vi "Sub-VI_Erros-Soma-Sensores.vi"(0 "Boolean 2":bool, 1 "Boolean 3":bool, 2 "Boolean 9":bool, 3 "Boolean 6":bool, 4 "Boolean 4":bool, 5 "Boolean 5":bool, 6 "Boolean 7":bool, 7 "Boolean 8":bool) -> (14 "Boolean":bool)   [LabVIEW 2019]
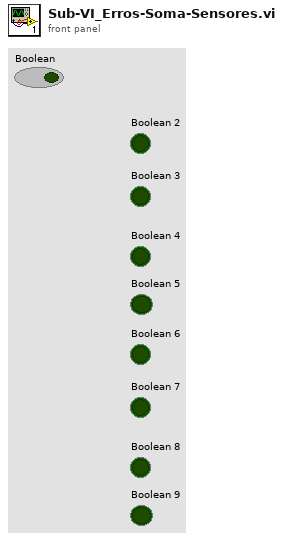
[diagram p1: front panel]
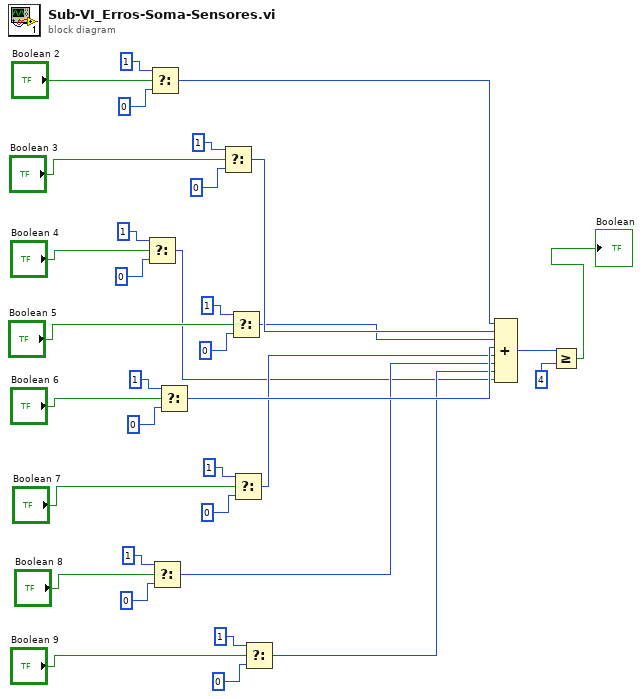
[diagram p0: block diagram]
diagram:
  n1 = Select(t=1, s="Boolean 4", f=0) -> (s? t:f=w1:i32)
  n2 = Select(t=1, s="Boolean 2", f=0) -> (s? t:f=w8:i32)
  n3 = Select(t=1, s="Boolean 8", f=0) -> (s? t:f=w3:i32)
  n4 = Select(t=1, s="Boolean 6", f=0) -> (s? t:f=w5:i32)
  n5 = Select(t=1, s="Boolean 3", f=0) -> (s? t:f=w7:i32)
  n6 = Select(t=1, s="Boolean 5", f=0) -> (s? t:f=w6:i32)
  n7 = Select(t=1, s="Boolean 7", f=0) -> (s? t:f=w4:i32)
  n8 = Select(t=1, s="Boolean 9", f=0) -> (s? t:f=w2:i32)
  n9 = Compound Arithmetic op=ADD(w8, w7, w6, w5, w4, w3, w2, w1) -> (w35:i32)
  n10 = Greater Or Equal?(x=w35, y=4) -> (x >= y?=→"Boolean":bool)
